vi "2 Ball Double Hot Half.vi"(1 "Run?":bool) -> (0 "Done?":bool)   [LabVIEW 2013]
uses:
  Globals/Homes.vi
  Globals/Useful Values.vi
panel:
  out "The Vision":dbl
  out "Sum":dbl
  out "Ready for Vision?":bool
  out "Time Elapsed":dbl
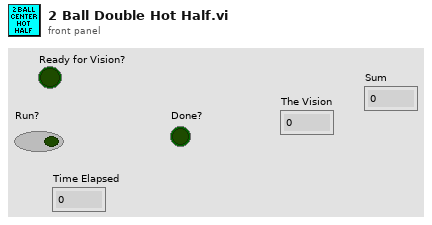
[diagram p1: front panel]
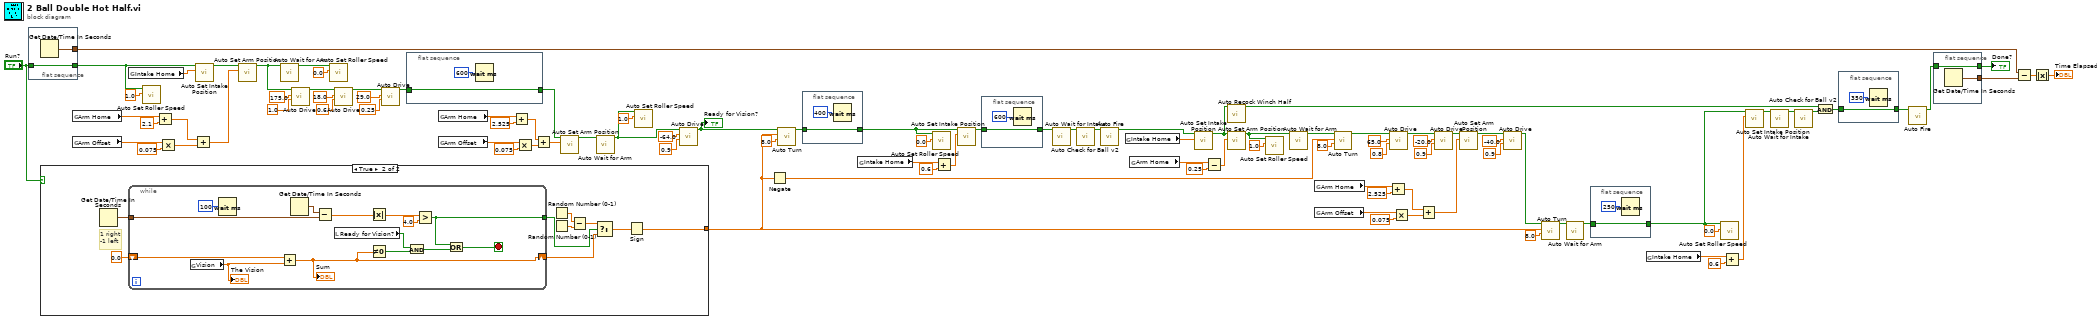
[diagram p0: block diagram]
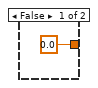
[diagram p2: hidden frame]
diagram:
  n1 = flat-sequence {
    tunnel: "Run?" -> [w101]
    tunnel: [w101] -> w25
    tunnel: [w100] -> w58
    frame #0 {
      n2 = Get Date/Time In Seconds() -> (seconds since 1Jan1904=w100:timestamp)
    }
  }
  n3 = case shown="True" "Run?" {
    tunnel: [0.0 w103] -> w3
    frame False {
    }
    frame True {
      # "1 right\n-1 left"
      n4 = Get Date/Time In Seconds() -> (seconds since 1Jan1904=w110:timestamp)
      n5 = while {
        shift-right: [w121] -> w105
        shift-left: 0.0 -> [w124]
        tunnel: w110 -> [w119]
        tunnel: [w112] -> w106
        stop <- w114 stop-if-true
        n6 = global read "Useful Values.vi" "Vision"() -> (w125:dbl)
        "The Vision" <- w125
        n7 = Wait (ms)(milliseconds to wait=u32 100) -> ()  [unwired: 1 out]
        n8 = Add(x=w124, y=w125) -> (x+y=w121:dbl)
        "Sum" <- w121
        n9 = Get Date/Time In Seconds() -> (seconds since 1Jan1904=w118:timestamp)
        n10 = Subtract(x=w118, y=w119) -> (x-y=w117:dbl)
        n11 = local read "Ready for Vision?"() -> (w122:bool)
        n12 = Absolute Value(x=w117) -> (abs(x)=w116:dbl)
        n13 = Not Equal To 0?(x=w121) -> (x != 0?=w120:bool)
        n14 = And(x=w122, y=w120) -> (x .and. y?=w113:bool)
        n15 = Greater?(x=w116, y=4.0) -> (0:w112:bool)
        n16 = Or(x=w112, y=w113) -> (x .or. y?=w114:bool)
      }
      n17 = Random Number (0-1)() -> (number: 0 to 1=w107:dbl)
      n18 = Random Number (0-1)() -> (number: 0 to 1=w108:dbl)
      n19 = Subtract(x=w107, y=w108) -> (x-y=w109:dbl)
      n20 = Select(t=w109, s=w106, f=w105) -> (s? t:f=w104:dbl)
      n21 = Sign(1:w104) -> (0:w103:dbl)
    }
  }
  n22 = global read "Homes.vi" "Arm Home"() -> (w98:dbl)
  n23 = global read "Useful Values.vi" "Arm Offset"() -> (w94:dbl)
  n24 = global read "Homes.vi" "Intake Home"() -> (w97:dbl)
  n25 = call "Auto Set Roller Speed.vi"("Value"=1.0, "Run?"=w25) -> ()  [unwired: 9 in, 1 out]
  n26 = Add(x=w98, y=2.1) -> (x+y=w93:dbl)
  n27 = Multiply(x=w94, y=0.075) -> (x*y=w96:dbl)
  n28 = Add(x=w93, y=w96) -> (x+y=w7:dbl)
  n29 = call "Auto Set Intake Position.vi"("Intake Position"=w97, "Run?"=w25) -> ("Done"=w6:bool)  [unwired: 9 in]
  n30 = call "Auto Set Arm Position.vi"("Arm Position"=w7, "Run?"=w6) -> ("Done"=w5:bool)  [unwired: 9 in]
  n31 = call "Auto Wait for Arm.vi"("Run?"=w5) -> ("Done"=w4:bool)  [unwired: 10 in]
  n32 = call "Auto Drive.vi"("Speed"=1.0, "Amount"=175.0, "Run?"=w5) -> ("Done"=w13:bool)  [unwired: 8 in]
  n33 = call "Auto Set Roller Speed.vi"("Value"=0.0, "Run?"=w4) -> ()  [unwired: 9 in, 1 out]
  n34 = call "Auto Drive.vi"("Speed"=0.6, "Amount"=18.0, "Run?"=w13) -> ("Done"=w12:bool)  [unwired: 8 in]
  n35 = call "Auto Drive.vi"("Speed"=0.25, "Amount"=29.0, "Run?"=w12) -> ("Done"=w35:bool)  [unwired: 8 in]
  n36 = flat-sequence {
    tunnel: w35 -> [w126]
    tunnel: [w126] -> w75
    frame #0 {
      n37 = Wait (ms)(milliseconds to wait=u32 600) -> ()  [unwired: 1 out]
    }
  }
  n38 = global read "Homes.vi" "Arm Home"() -> (w84:dbl)
  n39 = global read "Useful Values.vi" "Arm Offset"() -> (w89:dbl)
  n40 = Add(x=w84, y=2.525) -> (x+y=w90:dbl)
  n41 = Multiply(x=w89, y=0.075) -> (x*y=w87:dbl)
  n42 = Add(x=w90, y=w87) -> (x+y=w85:dbl)
  n43 = call "Auto Set Arm Position.vi"("Arm Position"=w85, "Run?"=w75) -> ("Done"=w83:bool)  [unwired: 9 in]
  n44 = call "Auto Wait for Arm.vi"("Run?"=w83) -> ("Done"=w26:bool)  [unwired: 10 in]
  n45 = call "Auto Set Roller Speed.vi"("Value"=1.0, "Run?"=w26) -> ()  [unwired: 9 in, 1 out]
  n46 = call "Auto Drive.vi"("Speed"=0.9, "Amount"=-64.0, "Run?"=w26) -> ("Done"=w1:bool)  [unwired: 8 in]
  "Ready for Vision?" <- w1
  n47 = Negate(x=w3) -> (-x=w55:dbl)
  n48 = call "Auto Turn.vi"("Turn Amount"=8.0 ("+/-?"), "+/-?"=w3, "Run?"=w1) -> ("Done"=w38:bool)  [unwired: 8 in]
  n49 = flat-sequence {
    tunnel: [w128] -> w27
    tunnel: w38 -> [w128]
    frame #0 {
      n50 = Wait (ms)(milliseconds to wait=u32 400) -> ()  [unwired: 1 out]
    }
  }
  n51 = global read "Homes.vi" "Intake Home"() -> (w54:dbl)
  n52 = call "Auto Set Roller Speed.vi"("Value"=0.0, "Run?"=w27) -> ()  [unwired: 9 in, 1 out]
  n53 = Add(x=w54, y=0.6) -> (x+y=w52:dbl)
  n54 = call "Auto Set Intake Position.vi"("Intake Position"=w52, "Run?"=w27) -> ("Done"=w39:bool)  [unwired: 9 in]
  n55 = flat-sequence {
    tunnel: [w130] -> w40
    tunnel: w39 -> [w130]
    frame #0 {
      n56 = Wait (ms)(milliseconds to wait=u32 600) -> ()  [unwired: 1 out]
    }
  }
  n57 = call "Auto Wait for Intake.vi"("Run?"=w40) -> ("Done"=w47:bool)  [unwired: 10 in]
  n58 = call "Auto Check for Ball v2.vi"("Run?"=w47) -> ("Done"=w74:bool)  [unwired: 10 in]
  n59 = call "Auto Fire.vi"("Run?"=w74) -> ("Done"=w45:bool)  [unwired: 10 in]
  n60 = global read "Homes.vi" "Intake Home"() -> (w43:dbl)
  n61 = global read "Homes.vi" "Arm Home"() -> (w73:dbl)
  n62 = call "Auto Set Intake Position.vi"("Intake Position"=w43, "Run?"=w45) -> ("Done"=w44:bool)  [unwired: 9 in]
  n63 = Subtract(x=w73, y=0.25) -> (x-y=w71:dbl)
  n64 = call "Auto Recock Winch Half.vi"("Run?"=w44) -> ("Done"=w61:bool)  [unwired: 10 in]
  n65 = call "Auto Set Arm Position.vi"("Arm Position"=w71, "Run?"=w44) -> ("Done"=w28:bool)  [unwired: 9 in]
  n66 = call "Auto Set Roller Speed.vi"("Value"=1.0, "Run?"=w28) -> ()  [unwired: 9 in, 1 out]
  n67 = call "Auto Wait for Arm.vi"("Run?"=w28) -> ("Done"=w37:bool)  [unwired: 10 in]
  n68 = global read "Homes.vi" "Arm Home"() -> (w69:dbl)
  n69 = global read "Useful Values.vi" "Arm Offset"() -> (w65:dbl)
  n70 = call "Auto Turn.vi"("Turn Amount"=8.0, "+/-?"=w55, "Run?"=w37) -> ("Done"=w30:bool)  [unwired: 8 in]
  n71 = call "Auto Drive.vi"("Speed"=0.8, "Amount"=65.0, "Run?"=w30) -> ("Done"=w9:bool)  [unwired: 8 in]
  n72 = Add(x=w69, y=2.525) -> (x+y=w64:dbl)
  n73 = Multiply(x=w65, y=0.075) -> (x*y=w67:dbl)
  n74 = Add(x=w64, y=w67) -> (x+y=w63:dbl)
  n75 = call "Auto Drive.vi"("Speed"=0.9, "Amount"=-20.0, "Run?"=w9) -> ("Done"=w8:bool)  [unwired: 8 in]
  n76 = call "Auto Set Arm Position.vi"("Arm Position"=w63, "Run?"=w8) -> ("Done"=w16:bool)  [unwired: 9 in]
  n77 = call "Auto Drive.vi"("Speed"=0.9, "Amount"=-40.0, "Run?"=w16) -> ("Done"=w31:bool)  [unwired: 8 in]
  n78 = call "Auto Turn.vi"("Turn Amount"=8.0, "+/-?"=w3, "Run?"=w31) -> ("Done"=w19:bool)  [unwired: 8 in]
  n79 = call "Auto Wait for Arm.vi"("Run?"=w19) -> ("Done"=w18:bool)  [unwired: 10 in]
  n80 = flat-sequence {
    tunnel: w18 -> [w132]
    tunnel: [w132] -> w17
    frame #0 {
      n81 = Wait (ms)(milliseconds to wait=u32 250) -> ()  [unwired: 1 out]
    }
  }
  n82 = global read "Homes.vi" "Intake Home"() -> (w48:dbl)
  n83 = call "Auto Set Roller Speed.vi"("Value"=0.0, "Run?"=w17) -> ()  [unwired: 9 in, 1 out]
  n84 = Add(x=w48, y=0.6) -> (x+y=w50:dbl)
  n85 = call "Auto Set Intake Position.vi"("Intake Position"=w50, "Run?"=w17) -> ("Done"=w51:bool)  [unwired: 9 in]
  n86 = call "Auto Wait for Intake.vi"("Run?"=w51) -> ("Done"=w46:bool)  [unwired: 10 in]
  n87 = call "Auto Check for Ball v2.vi"("Run?"=w46) -> ("Done"=w62:bool)  [unwired: 10 in]
  n88 = And(x=w61, y=w62) -> (x .and. y?=w21:bool)
  n89 = flat-sequence {
    tunnel: w21 -> [w134]
    tunnel: [w134] -> w20
    frame #0 {
      n90 = Wait (ms)(milliseconds to wait=u32 350) -> ()  [unwired: 1 out]
    }
  }
  n91 = call "Auto Fire.vi"("Run?"=w20) -> ("Done"=w29:bool)  [unwired: 10 in]
  n92 = flat-sequence {
    tunnel: w29 -> [w137]
    tunnel: [w137] -> w60
    tunnel: [w136] -> w59
    frame #0 {
      n93 = Get Date/Time In Seconds() -> (seconds since 1Jan1904=w136:timestamp)
    }
  }
  n94 = Subtract(x=w58, y=w59) -> (x-y=w57:dbl)
  n95 = Absolute Value(x=w57) -> (abs(x)=→"Time Elapsed":dbl)
  "Done?" <- w60
